vi "canver.vi"() -> (0 "子字符串":string)   [LabVIEW 2020]
uses:
  TEST1/ControlCAN/ControlCAN.llb/VCI_CAN_OBJ.ctl
  TEST1/ControlCAN/ControlCAN.llb/DevType.ctl
  TEST1/ControlCAN/ControlCAN.llb/VCI_INIT_CONFIG.ctl
  TEST1/ControlCAN/ControlCAN.llb/InitFlag.ctl
  TEST1/ControlCAN/ControlCAN.llb/Fliter.ctl
  TEST1/ControlCAN/ControlCAN.llb/Mode.ctl
  TEST1/ControlCAN/ControlCAN.lvlib
panel:
  out "Recieve":T1[](array[typedef])
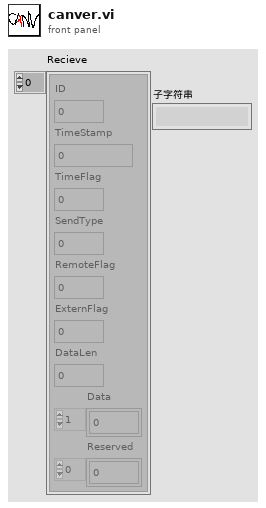
[diagram p1: front panel]
types:
  T1 = typedef "ControlCAN.lvlib/VCI_CAN_OBJ.ctl" = cluster{"ID":u32, "TimeStamp":u32, "TimeFlag":u8, "SendType":u8, "RemoteFlag":u8, "ExternFlag":u8, "DataLen":u8, "Data":u8[], "Reserved":u8[]}
  T2 = typedef "ControlCAN.lvlib/VCI_INIT_CONFIG.ctl" = cluster{"AccCode":u32, "AccMask":u32, "InitFlag":T3, "Fliter":T4, "Timing0":u8, "Timing1":u8, "Mode":T5}
  T3 = typedef "ControlCAN.lvlib/InitFlag.ctl" = u32
  T4 = typedef "ControlCAN.lvlib/Fliter.ctl" = u8
  T5 = typedef "ControlCAN.lvlib/Mode.ctl" = u8
  T6 = typedef "ControlCAN.lvlib/DevType.ctl" = u32
  T7 = cluster{"Recieve[0]":T1, "Recieve[1]":T1, "Recieve[2]":T1, "Recieve[3]":T1, "Recieve[4]":T1, "Recieve[5]":T1, "Recieve[6]":T1, "Recieve[7]":T1, "Recieve[8]":T1}
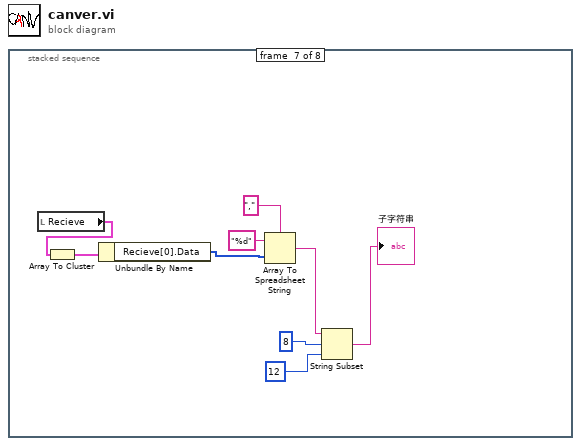
[diagram p0: block diagram]
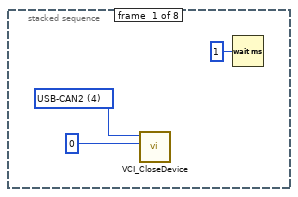
[diagram p2: hidden frame]
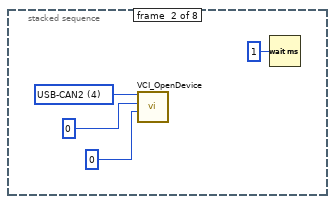
[diagram p3: hidden frame]
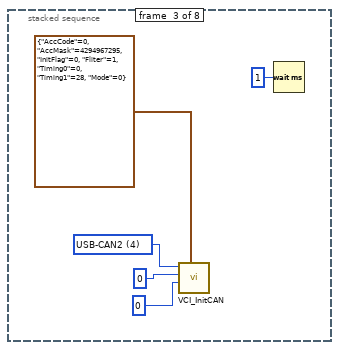
[diagram p4: hidden frame]
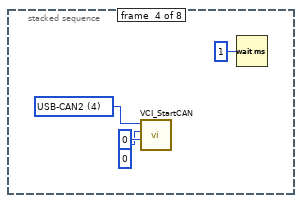
[diagram p5: hidden frame]
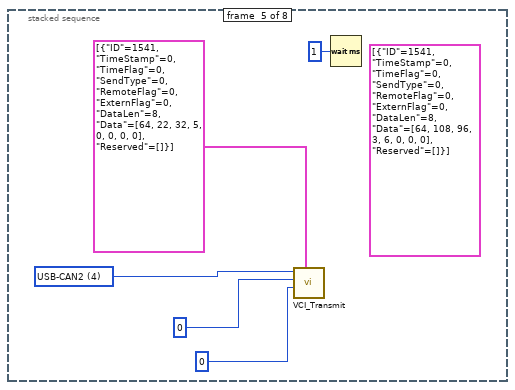
[diagram p6: hidden frame]
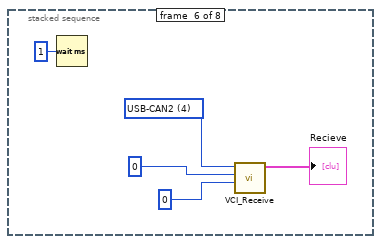
[diagram p7: hidden frame]
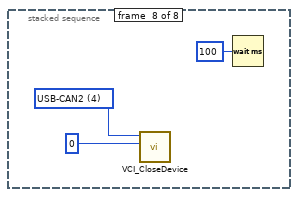
[diagram p8: hidden frame]
diagram:
  n1 = stacked-sequence {
    frame #0 {
      w3 = T6 4 items=["USB-CAN"=3, "USB-CAN2"=4] ("DevType")
      n2 = call "VCI_CloseDevice.vi"("DevIndex"=u32 0, "DevType"=w3) -> ()  [unwired: 8 in, 2 out]
      n3 = Wait (ms)(milliseconds to wait=u32 1 ("等待时间（毫秒）")) -> ()  [unwired: 1 out]
    }
    frame #1 {
      w5 = T6 4 items=["USB-CAN"=3, "USB-CAN2"=4] ("DevType")
      n4 = call "VCI_OpenDevice.vi"("Reserved"=u32 0, "DevIndex"=u32 0, "DevType"=w5) -> ()  [unwired: 7 in, 2 out]
      n5 = Wait (ms)(milliseconds to wait=u32 1 ("等待时间（毫秒）")) -> ()  [unwired: 1 out]
    }
    frame #2 {
      w9 = T6 4 items=["USB-CAN"=3, "USB-CAN2"=4] ("DevType")
      n6 = call "VCI_InitCAN.vi"("VCI_INIT_CONFIG"=T2 {"AccCode"=0, "AccMask"=4294967295, "InitFlag"=0, "Fliter"=1, "Timing0"=0, "Timing1"=28, "Mode"=0}, "CANIndex"=u32 0, "DevIndex"=u32 0, "DevType"=w9) -> ()  [unwired: 6 in, 2 out]
      n7 = Wait (ms)(milliseconds to wait=u32 1 ("等待时间（毫秒）")) -> ()  [unwired: 1 out]
    }
    frame #3 {
      w14 = T6 4 items=["USB-CAN"=3, "USB-CAN2"=4] ("DevType")
      n8 = call "VCI_StartCAN.vi"("CANIndex"=u32 0, "DevIndex"=u32 0, "DevType"=w14) -> ()  [unwired: 7 in, 2 out]
      n9 = Wait (ms)(milliseconds to wait=u32 1 ("等待时间（毫秒）")) -> ()  [unwired: 1 out]
    }
    frame #4 {
      (unwired) T1[] [{"ID"=1541, "TimeStamp"=0, "TimeFlag"=0, "SendType"=0, "RemoteFlag"=0, "ExternFlag"=0, "DataLen"=8, "Data"=[64, 108, 96, 3, 6, 0, 0, 0], "Reserved"=[]}] ("Buffer")
      w19 = T6 4 items=["USB-CAN"=3, "USB-CAN2"=4] ("DevType")
      n10 = call "VCI_Transmit.vi"("Buffer"=T1[] [{"ID"=1541, "TimeStamp"=0, "TimeFlag"=0, "SendType"=0, "RemoteFlag"=0, "ExternFlag"=0, "DataLen"=8, "Data"=[64, 22, 32, 5, 0, 0, 0, 0], "Reserved"=[]}], "CANIndex"=u32 0, "DevIndex"=u32 0, "DevType"=w19) -> ()  [unwired: 6 in, 2 out]
      n11 = Wait (ms)(milliseconds to wait=u32 1 ("等待时间（毫秒）")) -> ()  [unwired: 1 out]
    }
    frame #5 {
      w26 = T6 4 items=["USB-CAN"=3, "USB-CAN2"=4] ("DevType")
      n12 = Wait (ms)(milliseconds to wait=u32 1 ("等待时间（毫秒）")) -> ()  [unwired: 1 out]
      n13 = call "VCI_Receive.vi"("CANIndex"=u32 0, "DevIndex"=u32 0, "DevType"=w26) -> ("Recieve"=→"Recieve":T1[])  [unwired: 7 in, 1 out]
    }
    frame #6 {
      n14 = local read "Recieve"() -> (w33:T1[])
      n15 = Array To Cluster(array=w33) -> (cluster=w34:T7)
      n16 = Unbundle By Name(w34) -> ("Recieve[0].Data"=w35:u8[])
      n17 = Array To Spreadsheet String(delimiter (Tab)="," ("分隔符(Tab)"), array=w35, 3:"%d" ("格式字符串")) -> (spreadsheet string=w30:string)
      n18 = String Subset(string=w30, offset (0)=8 ("偏移量(0)"), length (rest)=12 ("长度（剩余）")) -> (substring=→"子字符串":string)
    }
    frame #7 {
      w38 = T6 4 items=["USB-CAN"=3, "USB-CAN2"=4] ("DevType")
      n19 = call "VCI_CloseDevice.vi"("DevIndex"=u32 0, "DevType"=w38) -> ()  [unwired: 8 in, 2 out]
      n20 = Wait (ms)(milliseconds to wait=u32 100 ("等待时间（毫秒）")) -> ()  [unwired: 1 out]
    }
  }
